vi "RealRootSolverMG.vi"() -> ()   [LabVIEW 2012]
doc: "VI calls in SubVI's that use the quadtratic formulas to solve the real roots."
panel:
  out "Imaginary x2":bool
  out "Imaginary x1":bool
  in  "stop":bool
  out "x2":dbl
  out "x1":dbl
  in  "c":dbl
  in  "b":dbl
  in  "a":dbl
  # "Marco Gonzalez\nEA 3\n03 / 02 / 2017"
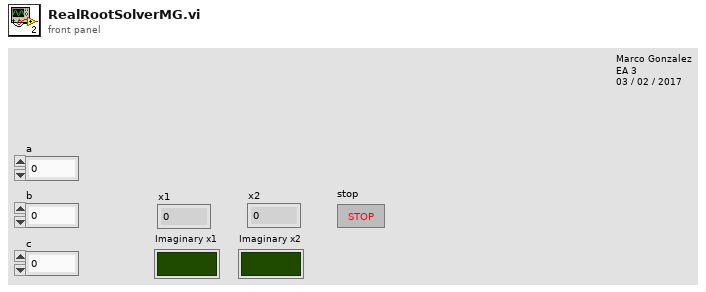
[diagram p1: front panel]
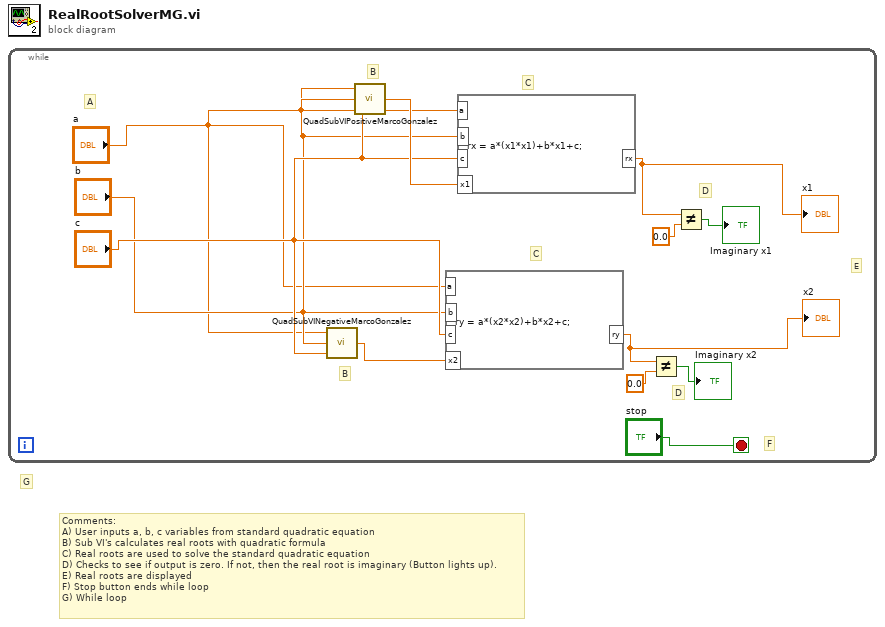
[diagram p0: block diagram]
diagram:
  # "G"
  # "Comments:\nA) User inputs a, b, c variables from standard quadratic equation\nB) Sub VI's calculates real roots with quadratic formula\nC) Real roots are used to solve the standard quadratic equation\nD) Checks to see if output is zero. If not, then the real root is imaginary (Button lights up).\nE) Real roots are displayed \nF) Stop button ends while loop\nG) While loop"
  n1 = while {
    stop <- "stop" stop-if-true
    # "F"
    # "E"
    # "D"
    # "D"
    # "C"
    # "C"
    # "B"
    # "B"
    # "A"
    n2 = call "QuadSubVINegativeMarcoGonzalez.vi"("c"="c", "b"="b", "a"="a") -> ("x2"=w10:dbl)
    n3 = call "QuadSubVIPositiveMarcoGonzalez.vi"("c"="c", "b"="b", "a"="a") -> ("x1"=w11:dbl)
    n4 = formula code="ry = a*(x2*x2)+b*x2+c;"("a"="a", "b"="b", "c"="c", "x2"=w10) -> ("ry"=w1:dbl)
    "x2" <- w1
    n5 = formula code="rx = a*(x1*x1)+b*x1+c;"("a"="a", "b"="b", "c"="c", "x1"=w11) -> ("rx"=w4:dbl)
    "x1" <- w4
    n6 = Not Equal?(x=w1, y=0.0) -> (x != y?=→"Imaginary x2":bool)
    n7 = Not Equal?(x=w4, y=0.0) -> (x != y?=→"Imaginary x1":bool)
  }
